vi "Launcher.vi"() -> ()   [LabVIEW 2016]
uses:
  APIs/Get/GetVI/GetVIByPath.vi
  APIs/Stimulus/VI/RunVI.vi
  APIs/Stimulus/VI/OpenVIFrontPanel.vi
  Drona.lvlib
  APIs/Get/GetVI/GetVI.lvlib
  apis/Stimulus/VI/VI.lvlib
panel:
  in  "Mode":string(combo)="Executable"
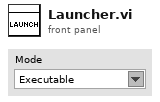
[diagram p1: front panel]
types:
  T1 = enum32{"Invalid", "Standard", "Closed", "Hidden", "Minimized", "Maximized"}
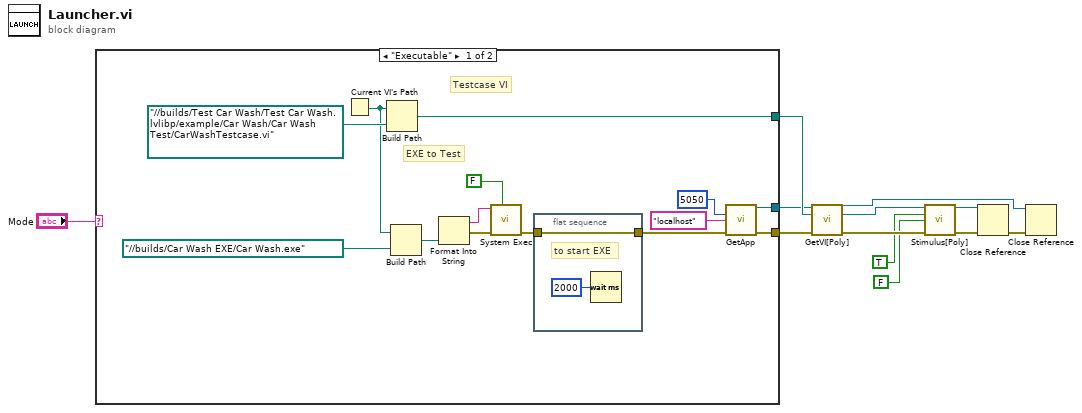
[diagram p0: block diagram]
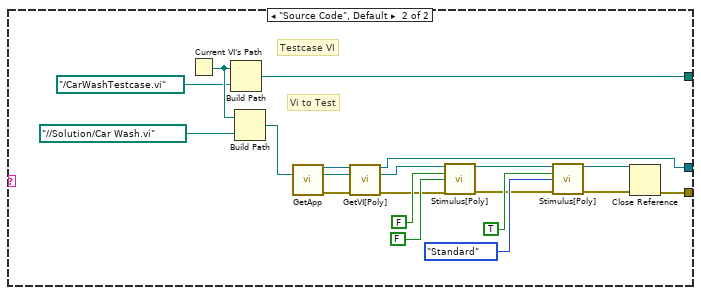
[diagram p2: hidden frame]
diagram:
  n1 = case shown="\"Executable\"" "Mode" {
    tunnel: [w25 w47] -> w10
    tunnel: [w15 w42] -> w8
    tunnel: [w13 w39] -> w7
    frame "Executable" {
      # "EXE to Test"
      # "Testcase VI"
      n2 = Current VI's Path() -> (path=w19:path)
      n3 = Build Path(base path=w19, name or relative path=path "../../builds/Test Car Wash/Test Car Wash.lvlibp/example/Car Wash/Car Wash Test/CarWashTestcase.vi" ("VI Path")) -> (appended path=w25:path)
      n4 = Build Path(base path=w19, name or relative path=path "../../builds/Car Wash EXE/Car Wash.exe" ("VI Name")) -> (appended path=w24:path)
      n5 = Format Into String(w24) -> (resulting string=w23:string, error out=w22:errorcluster)  [unwired: 3 in]
      n6 = call <vilib>:"System Exec.vi"("wait until completion? (T)"=FALSE, "error in (no error)"=w22, "command line"=w23) -> ("error out"=w20:errorcluster)  [unwired: 5 in, 3 out]
      n7 = flat-sequence {
        tunnel: [w28] -> w14
        tunnel: w20 -> [w28]
        frame #0 {
          # "to start EXE"
          n8 = Wait (ms)(milliseconds to wait=u32 2000) -> ()  [unwired: 1 out]
        }
      }
      n9 = call "GetApp.vi"("Port(0:Ignored)"=u16 5050, "Service Name (\"\":localhost)"="localhost" ("Project Name (\"\": ThisApplication)"), "error in (no error)"=w14) -> ("Application Ref"=w13:refnum<vi>, "error out"=w15:errorcluster)  [unwired: 11 in]
    }
    frame "Source Code", Default {
      # "Testcase VI"
      # "Vi to Test"
      n10 = Current VI's Path() -> (path=w46:path)
      n11 = Build Path(base path=w46, name or relative path=path "../CarWashTestcase.vi" ("VI Path")) -> (appended path=w47:path)
      n12 = Build Path(base path=w46, name or relative path=path "../../Solution/Car Wash.vi" ("VI Name")) -> (appended path=w43:path)
      n13 = call "GetApp.vi"() -> ("Application Ref"=w40:refnum<vi>, "error out"=w41:errorcluster)  [unwired: 14 in]
      n14 = call-poly "GetVI[Poly].vi"("Application Ref in"=w40, "VI Path"=w43, "error in (no error)"=w41) -> ("Application Ref out"=w39:refnum<vi>, "VI Reference"=w38:refnum<vi>, "error out"=w31:errorcluster)  [unwired: 10 in]
      n15 = call-poly "Stimulus[Poly].vi"("VI Reference In"=w38, "Wait Until Done (F)"=FALSE ("Wait Until Done"), "Auto Dispose Reference (F)"=FALSE ("Auto Dispose Reference"), "error in"=w31) -> ("VI Reference Out"=w35:refnum<vi>, "error out"=w32:errorcluster)  [unwired: 10 in]
      n16 = call-poly "Stimulus[Poly].vi"("VI Reference In"=w35, "Wait Until Done (F)"=TRUE ("Activate?"), "State(Standard)"=T1."Standard" ("State"), "error in"=w32) -> ("VI Reference Out"=w29:refnum<vi>, "error out"=w30:errorcluster)  [unwired: 10 in]
      n17 = Close Reference(reference=w29, error in (no error)=w30) -> (error out=w42:errorcluster)
    }
  }
  n18 = call-poly "GetVI[Poly].vi"("Application Ref in"=w7, "VI Path"=w10, "error in (no error)"=w8) -> ("Application Ref out"=w12:refnum<vi>, "VI Reference"=w4:refnum<vi>, "error out"=w6:errorcluster)  [unwired: 10 in]
  n19 = call-poly "Stimulus[Poly].vi"("VI Reference In"=w4, "Wait Until Done (F)"=TRUE ("Wait Until Done"), "Auto Dispose Reference (F)"=FALSE ("Auto Dispose Reference"), "error in"=w6) -> ("VI Reference Out"=w1:refnum<vi>, "error out"=w5:errorcluster)  [unwired: 10 in]
  n20 = Close Reference(reference=w1, error in (no error)=w5) -> (error out=w11:errorcluster)
  n21 = Close Reference(reference=w12, error in (no error)=w11) -> ()  [unwired: 1 out]
